vi "GrabToFrameQueue.vi"(5 "Enable multiple ROI? (F)":bool, 6 "Building ZLUT?":bool, 7 "ROI corner pos":cluster{"X":i32, "Y":i32}[](array[cluster]), 8 "Camera settings":T2={"Frame rate (Hz)"=50, "Gain [1-4]"=2.0, "Offset"=75, "Exposure time"=193, "Mode"=6, "ROIs"=[{"X"=24, "Y"=100}], "ROI Size"={"X"=200, "Y"=200}, "Number of buffers"=40, "ZLUT Gain"=1.0, "ZLUT exposure time"=1000, "Display framerate"=10, "Display image size"={"X"=1280, "Y"=1024}, "Use hardware multiple-ROI?"=FALSE} {"Exposure time" min=50}, 9 "Camera Out":refnum<queue>, 10 "Camera In":refnum<queue>, 11 "IMAQ Refnum":refnum<k11>) -> (3 "IMAQ Session Out":refnum<k11>)   [LabVIEW 2011]
uses:
  BeadTracker2.llb/Cmd_CameraIn.ctl
  BeadTracker2.llb/CmdEnum_CameraIn.ctl
  BeadTracker2.llb/CmdData_NewFrame.ctl
  <vilib>/vision/Image Controls.llb/IMAQ Image.ctl
  BeadTracker2.llb/CmdEnum_CameraFrameType.ctl
  CameraConfig.ctl
panel:
  out "Image":T1(plugin-control)
  in  "Display image?":bool
  out "Actual Width":u32
  # "us"
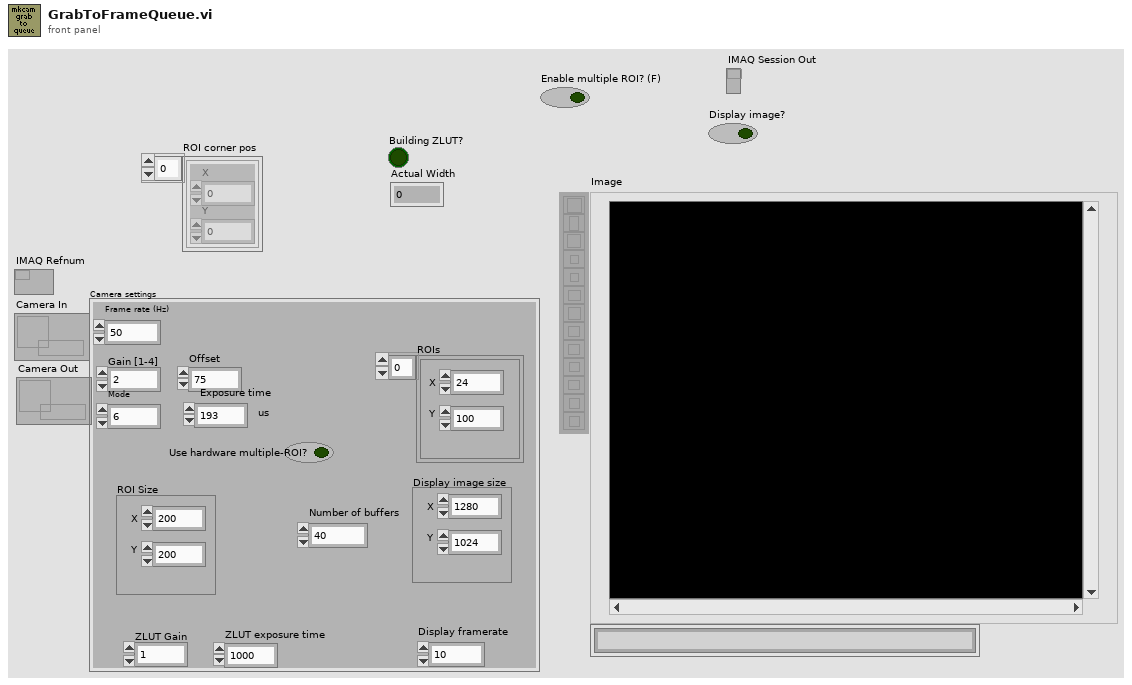
[diagram p1: front panel]
types:
  T1 = typedef "IMAQ Image.ctl" = refnum<image>
  T2 = typedef "CameraConfig.ctl" = cluster{"Frame rate (Hz)":u32, "Gain [1-4]":sgl, "Offset":i16, "Exposure time":i32, "Mode":i16, "ROIs":cluster{"X":i32, "Y":i32}[], "ROI Size":cluster{"X":i32, "Y":i32}, "Number of buffers":i32, "ZLUT Gain":sgl, "ZLUT exposure time":i32, "Display framerate":u32, "Display image size":cluster{"X":i32, "Y":i32}, "Use hardware multiple-ROI?":bool}
  T3 = typedef "CmdEnum_CameraFrameType.ctl" = enum16{"Full", "HardwareROI", "EndGrabMarker"}
  T4 = typedef "CmdData_NewFrame.ctl" = cluster{"Buffer Image":T1, "Frame #":i32, "Hardware ROI Index":i32, "Timestamp":dbl, "Type":T3}
  T5 = typedef "CmdEnum_CameraIn.ctl" = enum32{"Init", "Close", "ShowSettingsDialog", "EndGrab", "GrabZLUT", "GrabToTracker", "GrabToQueue", "AdjustROIs"}
  T6 = typedef "Cmd_CameraIn.ctl" = cluster{"ID":T5, "Msg Data":variant}
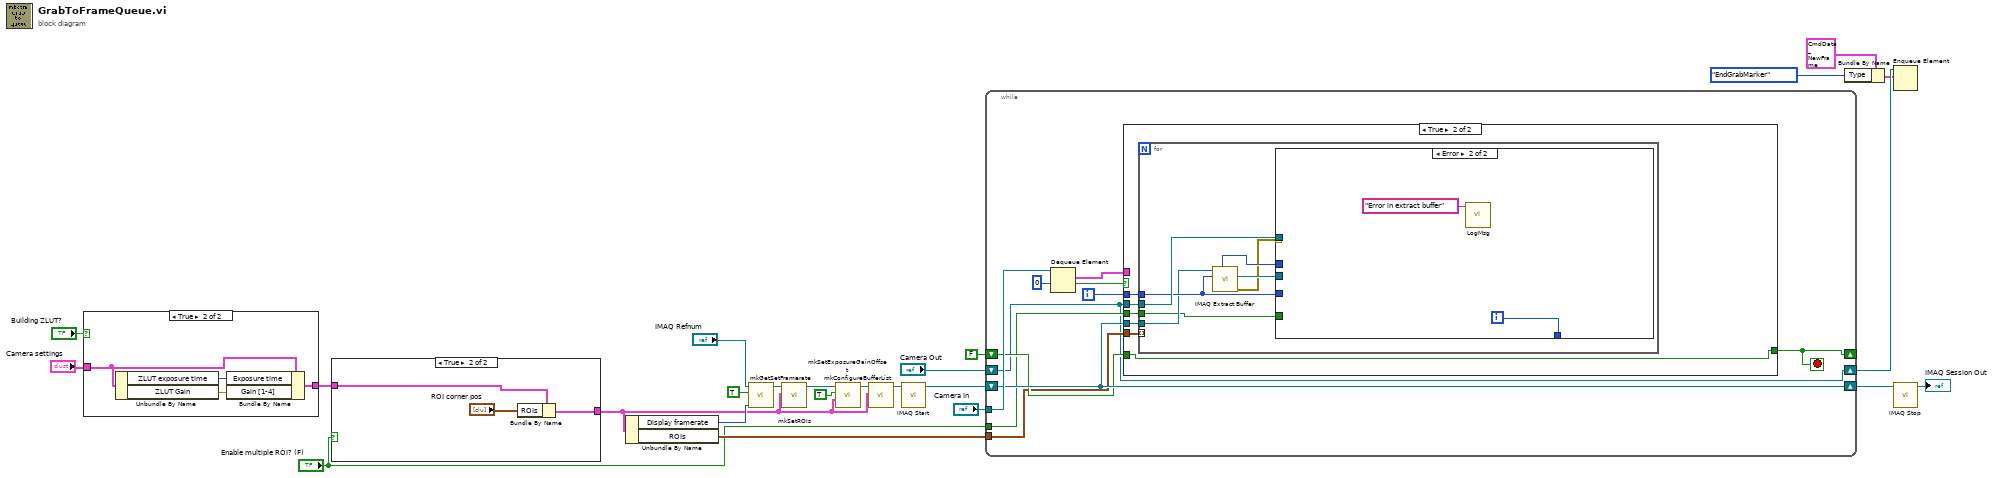
[diagram p0: block diagram]
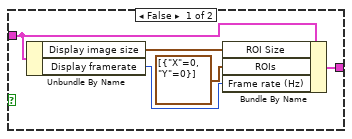
[diagram p3: hidden frame]
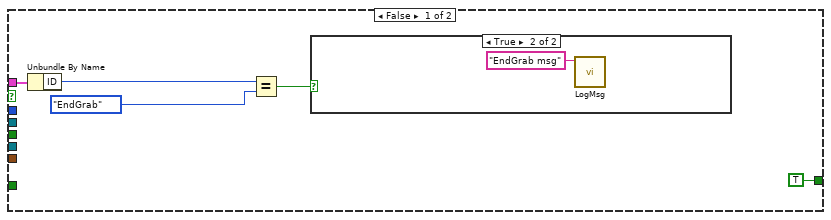
[diagram p4: hidden frame]
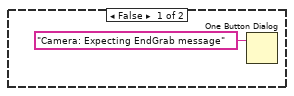
[diagram p5: hidden frame]
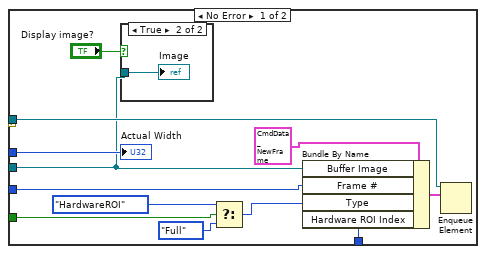
[diagram p6: hidden frame]
diagram:
  n1 = case shown="True" "Building ZLUT?" {
    tunnel: "Camera settings" -> [w25 w27]
    tunnel: [w25 w26] -> w11
    frame False {
    }
    frame True {
      n2 = Unbundle By Name(w27) -> ("ZLUT exposure time"=w29:i32, "ZLUT Gain"=w28:sgl)
      n3 = Bundle By Name(cluster=w27, "Exposure time"=w29, "Gain [1-4]"=w28) -> (w26:T2)
    }
  }
  n4 = case shown="True" "Enable multiple ROI? (F)" {
    tunnel: [w32 w37] -> w1
    tunnel: w11 -> [w30 w35]
    frame False {
      n5 = Unbundle By Name(w30) -> ("Display image size"=w34:cluster{"X":i32, "Y":i32}, "Display framerate"=w31:u32)
      n6 = Bundle By Name(cluster=w30, "ROI Size"=w34, "ROIs"=cluster{"X":i32, "Y":i32}[] [{"X"=0, "Y"=0}], "Frame rate (Hz)"=w31) -> (w32:T2)
    }
    frame True {
      n7 = Bundle By Name(cluster=w35, "ROIs"="ROI corner pos") -> (w37:T2)
    }
  }
  n8 = Unbundle By Name(w1) -> ("Display framerate"=w2:u32, "ROIs"=w18:cluster{"X":i32, "Y":i32}[])
  n9 = call "mkGetSetFramerate.vi"("Framerate"=w2, "Set? (F)"=TRUE, "IMAQ Refnum out"="IMAQ Refnum") -> ("IMAQ Refnum (out)"=w5:refnum<k11>)  [unwired: 5 in, 3 out]
  n10 = call "mkSetROIs.vi"("Camera in"=w1, "IMAQ Refnum in"=w5) -> ("IMAQ Refnum out"=w3:refnum<k11>)  [unwired: 9 in]
  n11 = call "mkSetExposureGainOffset.vi"("Camera settings (in)"=w1, "Set? (F)"=TRUE, "IMAQ Refnum in"=w3) -> ("IMAQ Refnum out"=w17:refnum<k11>)  [unwired: 5 in, 3 out]
  n12 = call "mkConfigureBufferList.vi"("Camera in"=w1, "IMAQ Session"=w17) -> ("IMAQ Session (out)"=w16:refnum<k11>)  [unwired: 9 in]
  n13 = call <vilib>:"IMAQ Start.vi"("IMAQ Session In"=w16) -> ("IMAQ Session Out"=w21:refnum<k11>)  [unwired: 9 in, 1 out]
  n14 = while {
    tunnel: "Camera In" -> [w48]
    shift-right: [w43] -> w20
    shift-left: w21 -> [w43]
    shift-right: [w39] -> _
    shift-left: FALSE ("stop") -> [w42]
    tunnel: "Enable multiple ROI? (F)" -> [w41]
    tunnel: w18 -> [w40]
    shift-right: [w38] -> w10
    shift-left: "Camera Out" -> [w38]
    i -> [w44]
    stop <- w39 stop-if-true
    n15 = Dequeue Element(queue=w48, timeout in ms (-1)=0) -> (element=w45:T6, timed out?=w47:bool)  [unwired: 1 in, 2 out]
    n16 = case shown="True" w47 {
      tunnel: w38 -> [_ w61]
      tunnel: w45 -> [w53 _]
      tunnel: w44 -> [_ w60]
      tunnel: w43 -> [_ w59]
      tunnel: [TRUE ("stop") w58] -> w39
      tunnel: w42 -> [_ w58]
      tunnel: w41 -> [_ w57]
      tunnel: w40 -> [_ w56]
      frame False {
        n17 = Unbundle By Name(w53) -> ("ID"=w52:T5)
        n18 = Equal?(x=w52, y=CmdEnum_CameraIn."EndGrab") -> (x = y?=w50:bool)
        n19 = case shown="True" w50 {
          frame False {
            n20 = One Button Dialog(message="Camera: Expecting EndGrab message") -> ()  [unwired: 1 in, 1 out]
          }
          frame True {
            n21 = call "LogMsg.vi"("msg"="EndGrab msg") -> ()  [unwired: 11 in]
          }
        }
      }
      frame True {
        n22 = for {
          tunnel: w61 -> [w69]
          tunnel: w60 -> [w68]
          tunnel: w59 -> [w67]
          tunnel: w57 -> [w63]
          tunnel: w56 -> [_] mode=indexing
          i -> [w64]
          n23 = call <vilib>:"IMAQ Extract Buffer.vi"("Buffer to extract"=w68, "IMAQ Session In"=w67) -> ("error out"=w62:errorcluster, "Image Out"=w65:T1, "Actual Width"=w66:u32)  [unwired: 4 in, 3 out]
          n24 = case shown="Error" w62 {
            tunnel: w69 -> [w79 _]
            tunnel: w68 -> [w78 _]
            tunnel: w66 -> [w77 _]
            tunnel: w65 -> [w75 _]
            tunnel: w64 -> [w74 _]
            tunnel: w63 -> [w73 _]
            frame No Error {
              n25 = case shown="True" "Display image?" {
                tunnel: w75 -> [_ w82]
                frame False {
                }
                frame True {
                  "Image" <- w82
                }
              }
              n26 = Select(t=CmdEnum_CameraFrameType."HardwareROI" ("Type"), s=w73, f=CmdEnum_CameraFrameType."Full") -> (s? t:f=w71:T3)
              n27 = Bundle By Name(cluster=T4 {"Buffer Image"=refnum, "Frame #"=0, "Hardware ROI Index"=0, "Timestamp"=0.0, "Type"=enum."Full"} ("Cluster"), "Buffer Image"=w75, "Frame #"=w78, "Type"=w71, "Hardware ROI Index"=w74) -> (w81:T4)
              n28 = Enqueue Element(queue=w79, element=w81) -> ()  [unwired: 2 in, 3 out]
              "Actual Width" <- w77
            }
            frame Error {
              n29 = call "LogMsg.vi"("msg"="Error in extract buffer") -> ()  [unwired: 11 in]
            }
          }
        }
      }
    }
  }
  n30 = Bundle By Name(cluster=T4 {"Buffer Image"=refnum, "Frame #"=0, "Hardware ROI Index"=0, "Timestamp"=0.0, "Type"=enum."Full"} ("Cluster"), "Type"=CmdEnum_CameraFrameType."EndGrabMarker" ("f")) -> (w7:T4)
  n31 = Enqueue Element(queue=w10, element=w7) -> ()  [unwired: 2 in, 3 out]
  n32 = call <vilib>:"IMAQ Stop.vi"("IMAQ Session In"=w20) -> ("IMAQ Session Out"=→"IMAQ Session Out":refnum<k11>)  [unwired: 9 in, 1 out]
